vi "SimpleLiveAppBufferIndexScrollBar.vi"() -> ()   [LabVIEW 2018]
uses:
  D:/SVN/PM/sdk/AppSamples/LabVIEWSamples/trunk/Release/2018/Dependencies/PVCamNET.dll
  Dependencies/PVCamNET.dll
panel:
  out "Buffer Index":dbl
  in  "Scroll bar":i32(c297)
  out "Capturing":bool
  in  "Exposure Time":dbl
  out "Live":bool
  out "Camera Status":bool
  in  "Uninit":bool
  in  "Live stop":bool
  in  "Live start":bool
  in  "Init":bool
  # "SimpleLiveAppBufferIndexScrollBar.vi\n\nDescription:\nThis sample code lets the user use live mode in an event driven structure.\nWhen live mode is paused the user is able to scroll the bar to view images.\n\nSteps to run:\n1. Click \"Run\"\n2. Click \"Open\"\n3. Enter Exposure Time\n4. Click \"Live start\"\n5. Click \"Live stop\"\n6.  Scroll the scroll bar\n7. Click \"Close\""
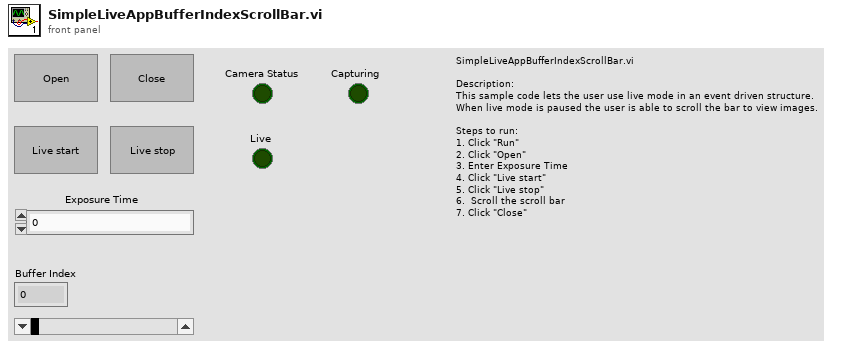
[diagram p1: front panel]
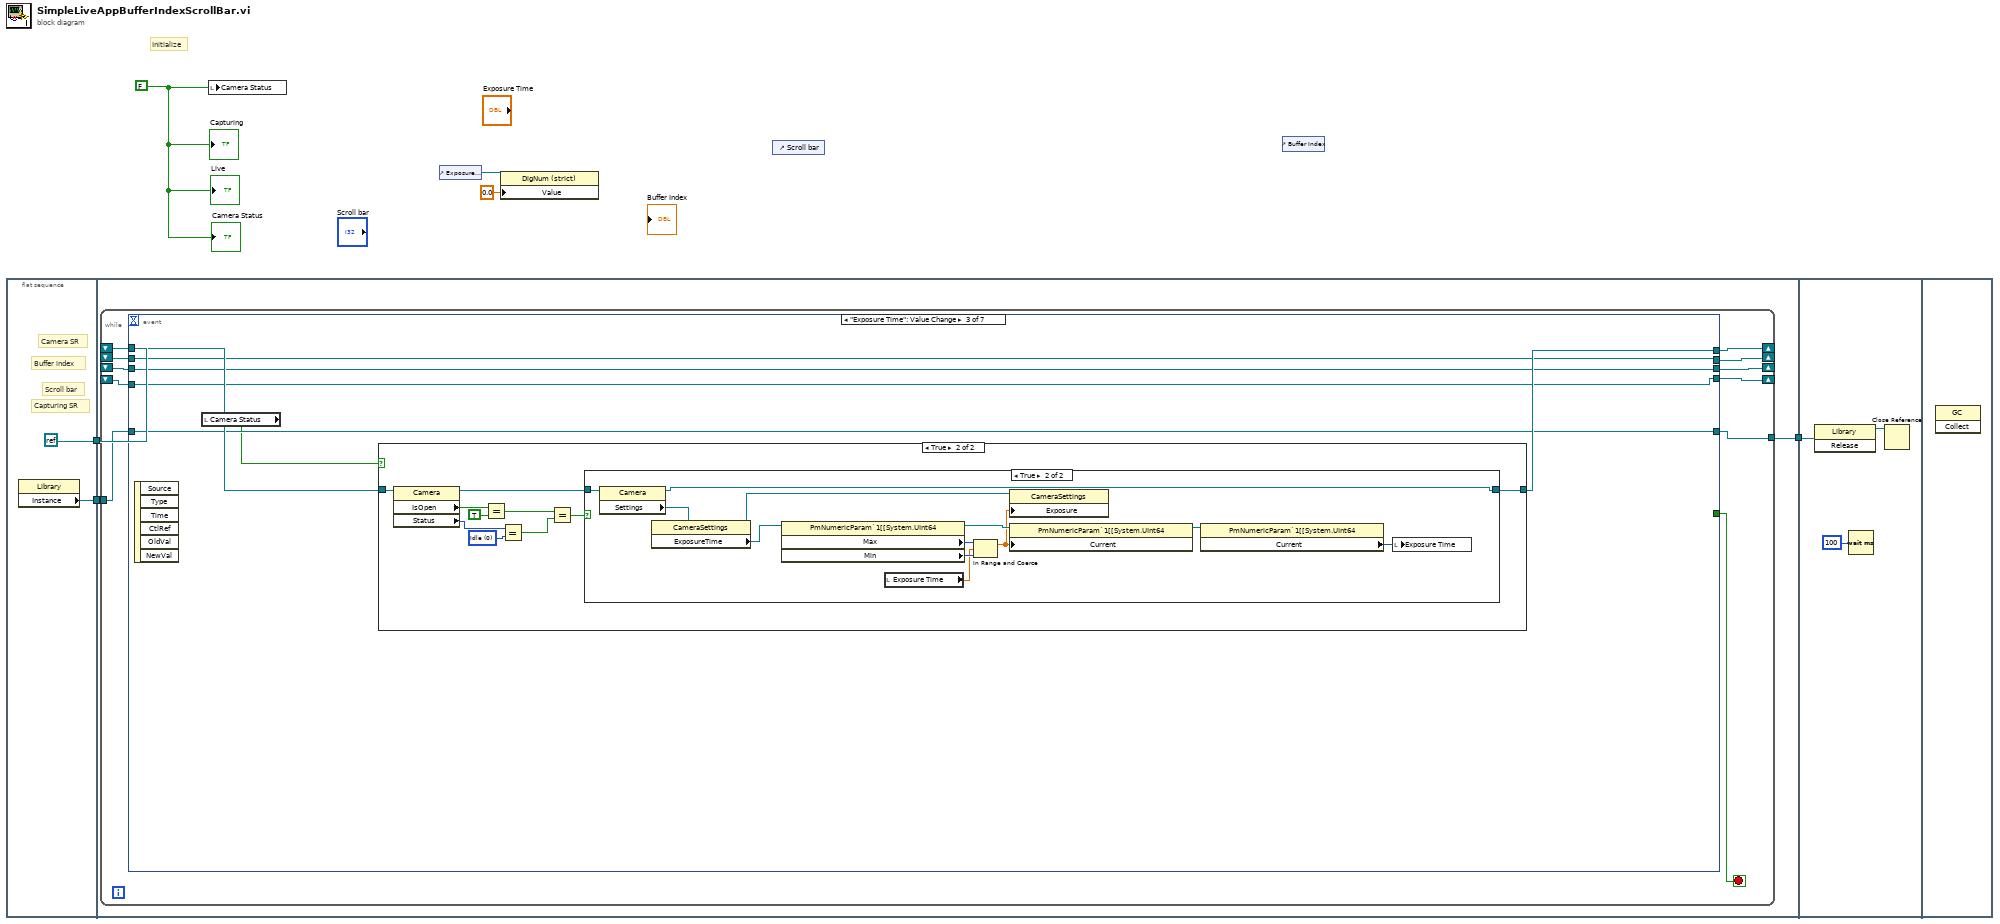
[diagram p0: block diagram]
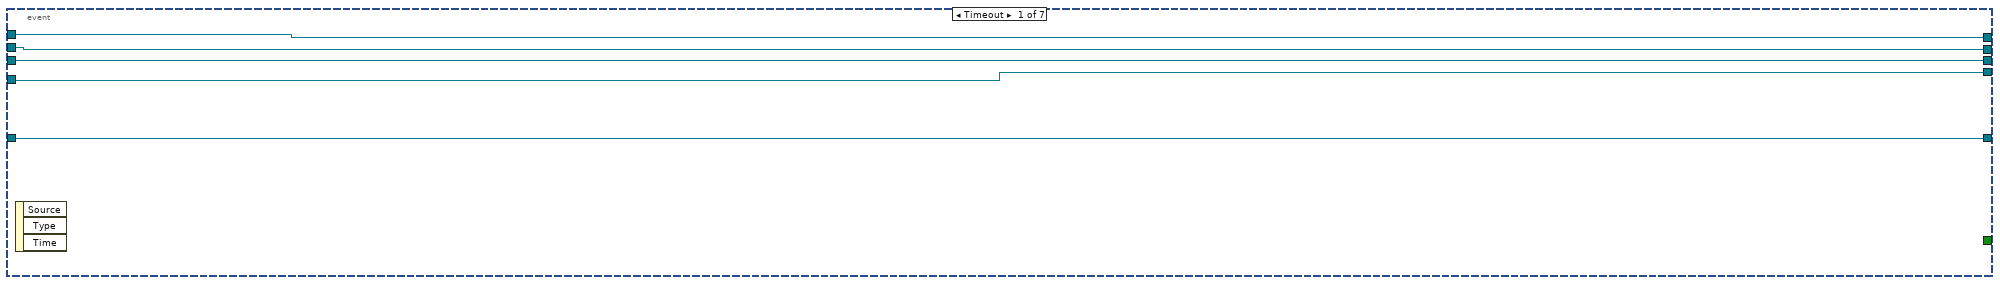
[diagram p2: hidden frame]
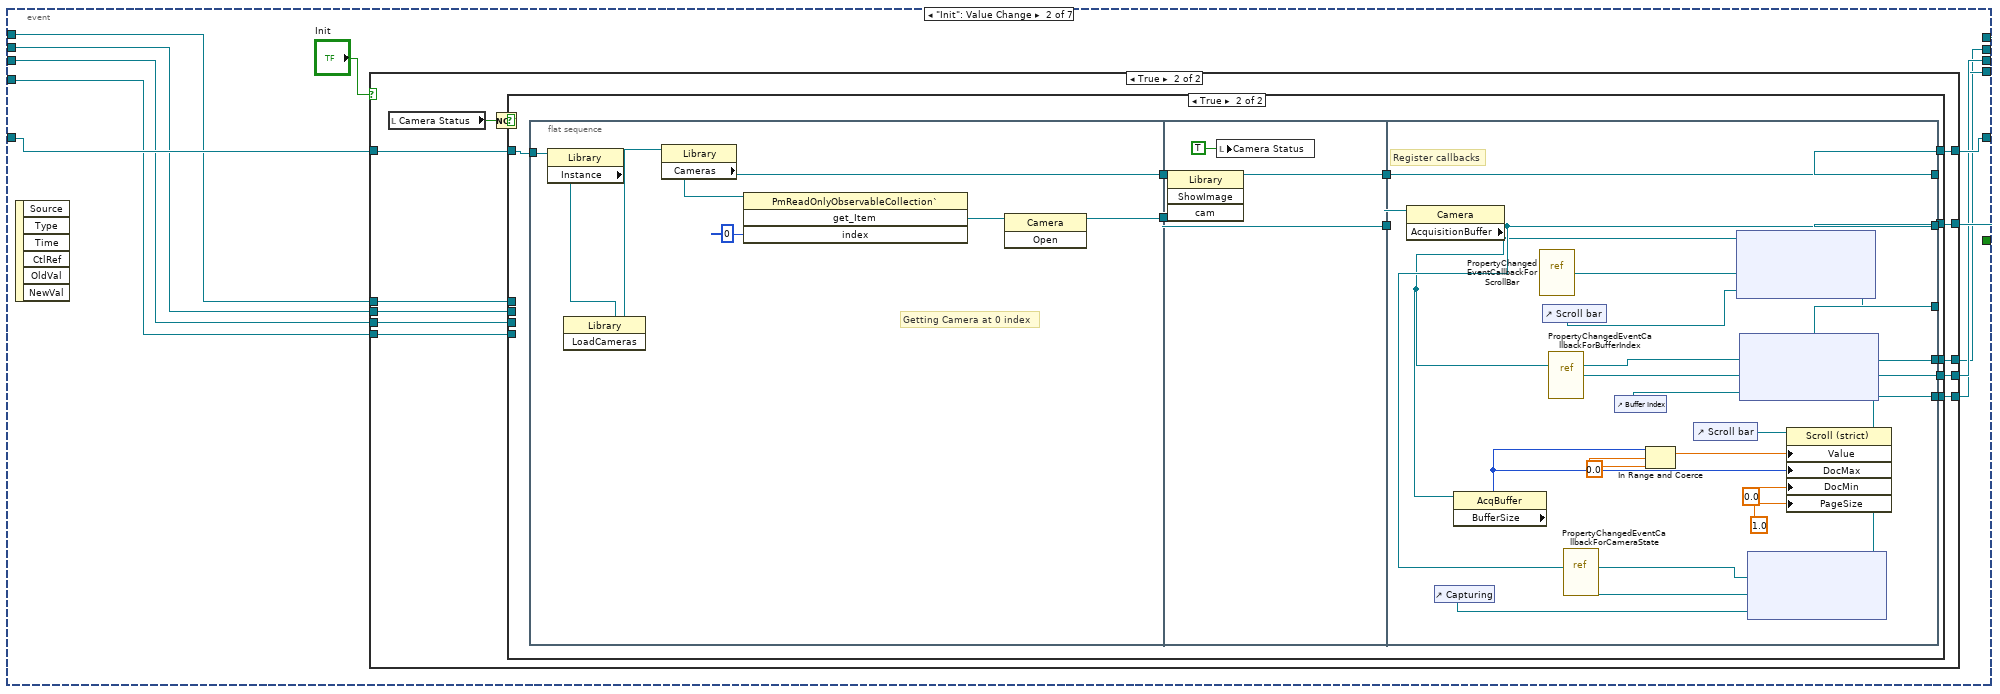
[diagram p3: hidden frame]
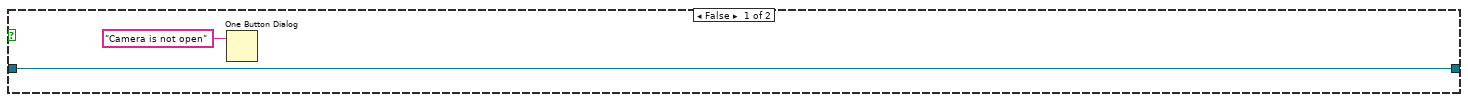
[diagram p6: hidden frame]
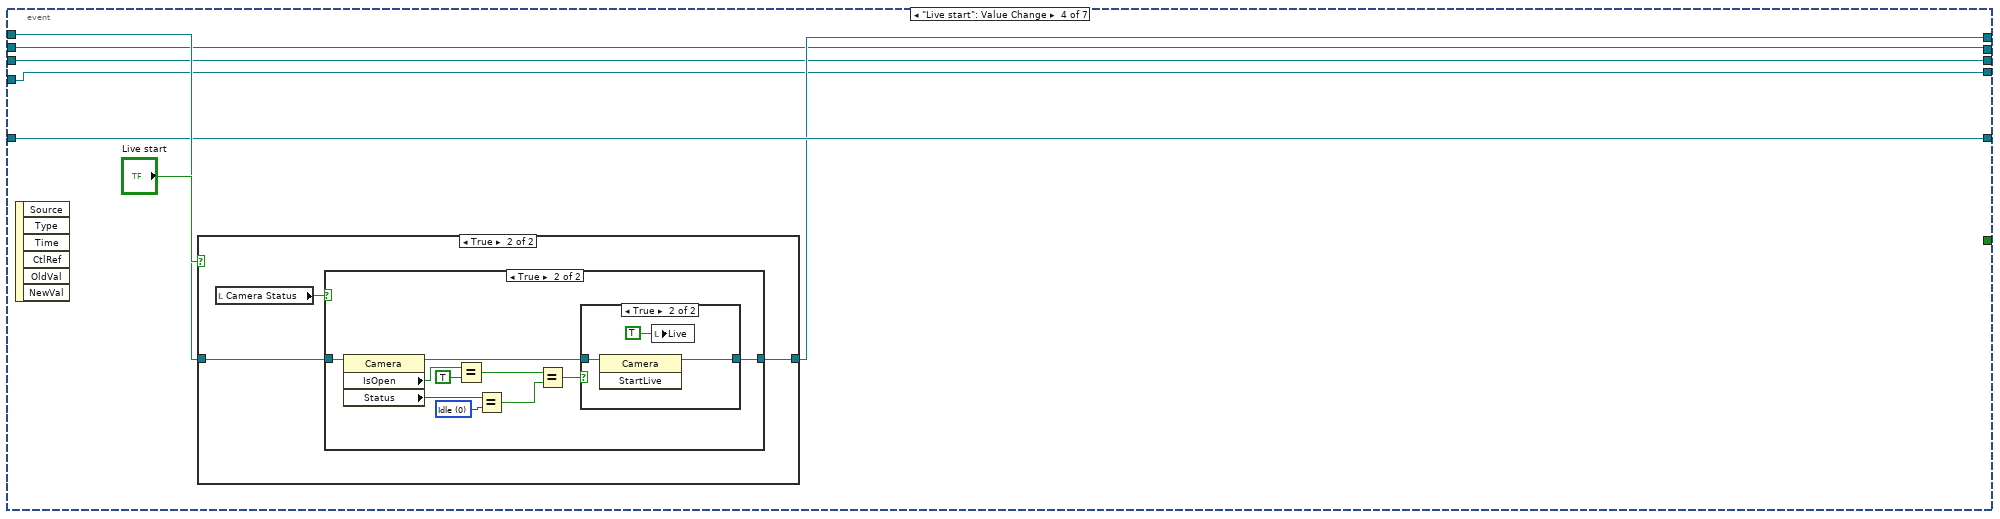
[diagram p8: hidden frame]
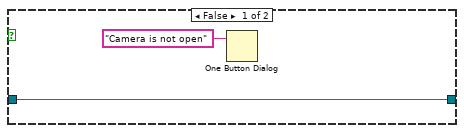
[diagram p10: hidden frame]
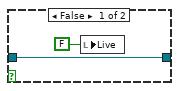
[diagram p11: hidden frame]
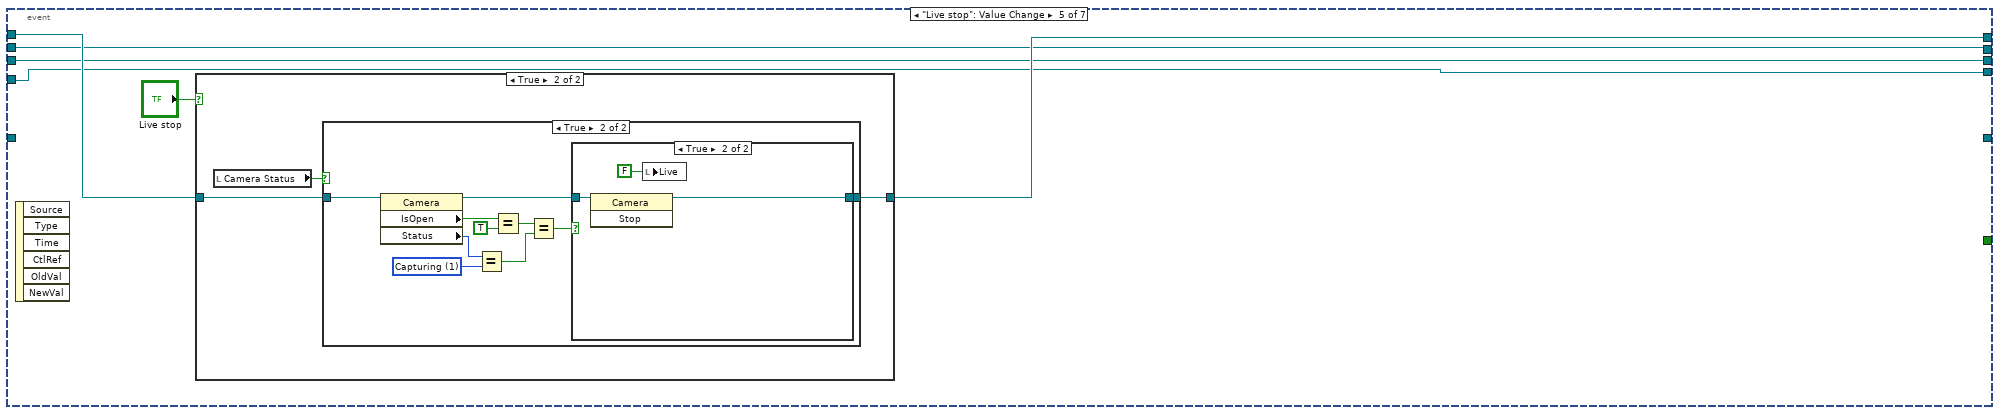
[diagram p12: hidden frame]
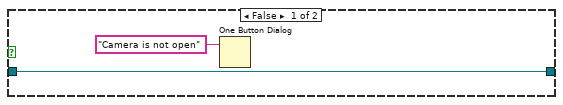
[diagram p14: hidden frame]
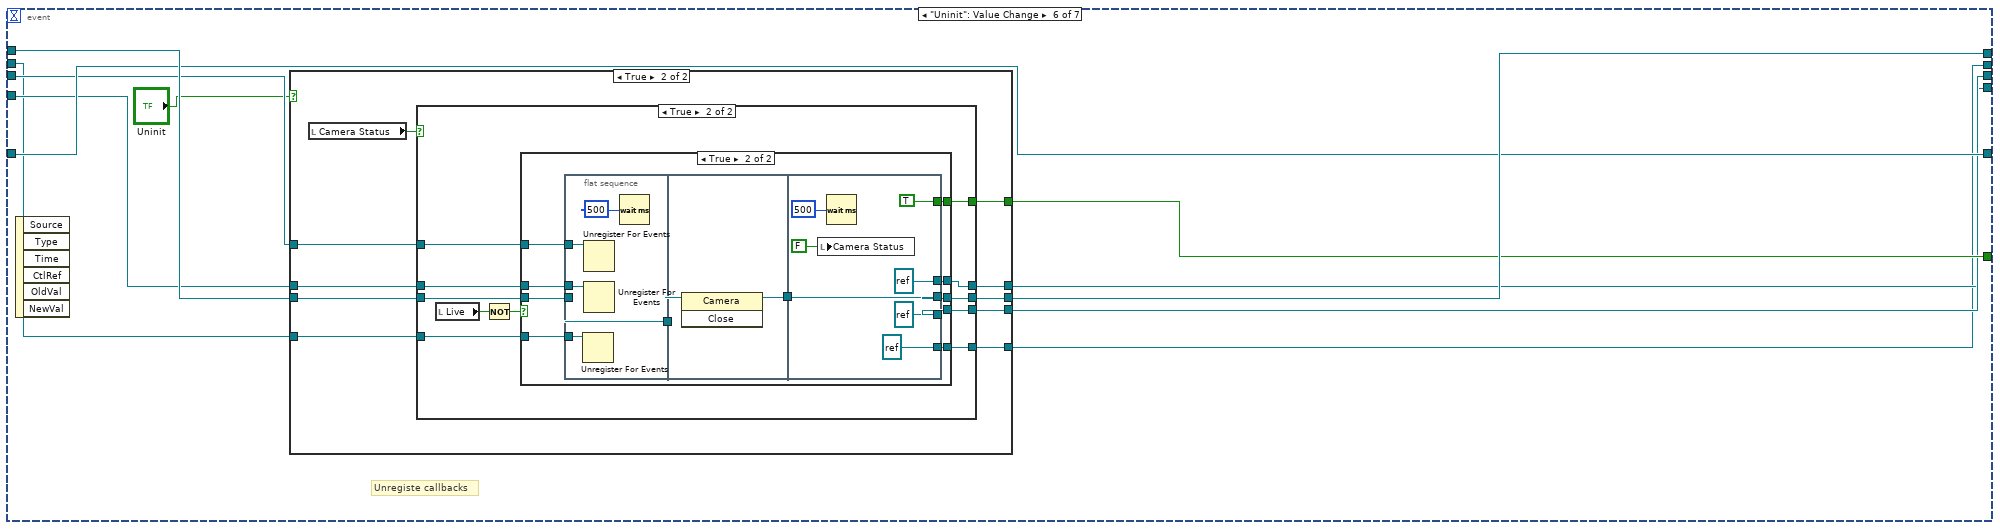
[diagram p16: hidden frame]
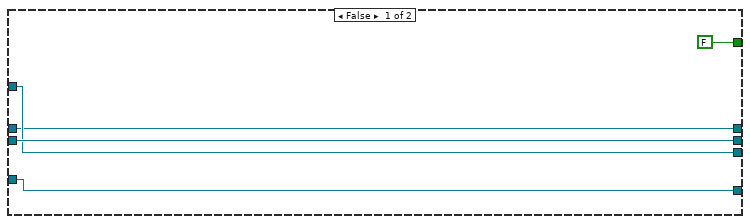
[diagram p17: hidden frame]
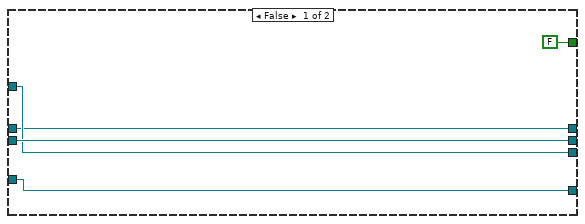
[diagram p18: hidden frame]
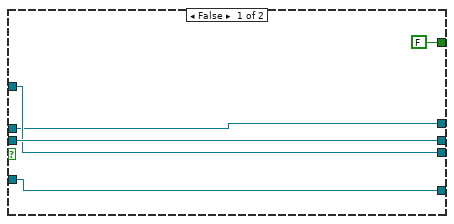
[diagram p19: hidden frame]
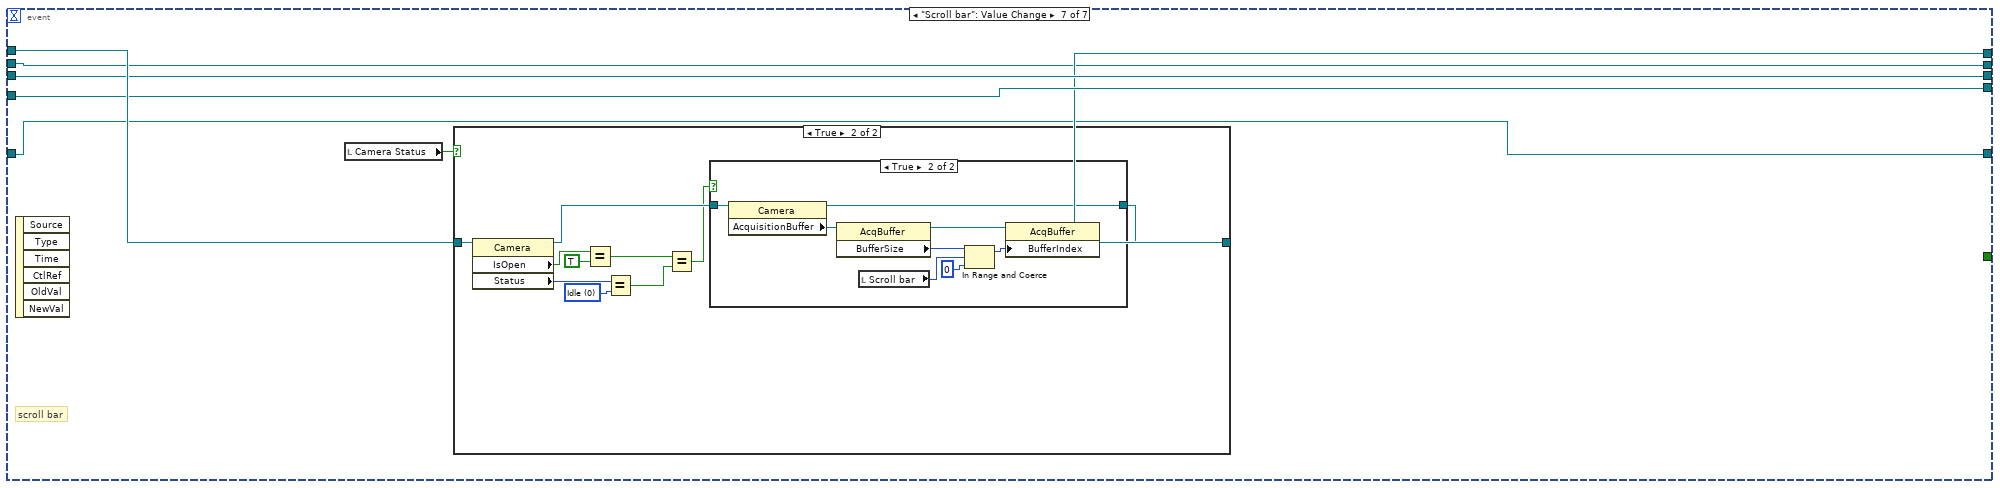
[diagram p20: hidden frame]
diagram:
  w3 = FALSE ("Histogram On/Off")
  # "Initialize"
  n1 = flat-sequence {
    tunnel: [w8] -> w6
    tunnel: [refnum<k0> refnum] -> w4
    tunnel: w6 -> [w11]
    tunnel: [w10] -> w5
    tunnel: w4 -> [w9]
    tunnel: w5 -> [w289]
    frame #0 {
      # "Buffer index"
      # "Capturing SR"
      # "Camera SR"
      # "Scroll bar"
      n2 = property class="Library"() -> ("Instance"=w8:refnum<k24>)  [unwired: 2 in, 2 out]
    }
    frame #1 {
      n3 = while {
        tunnel: w11 -> [w22]
        shift-right: [w21] -> _
        shift-left: w9 -> [w12]
        tunnel: [w20] -> w10
        shift-right: [w18] -> _
        shift-left: _ -> [w17]
        shift-right: [w16] -> _
        shift-left: _ -> [w15]
        shift-right: [w14] -> _
        shift-left: _ -> [w13]
        stop <- w19 stop-if-true
        n4 = event shown="[2] \"Exposure Time\": Value Change" {
          selector: _ -> [_ _ _ _ _ _ _]
          dyn-events: _ -> [_ _ _ _ _ _ _]
          timeout: _ -> [_ _ _ _ _ _ _]
          tunnel: w22 -> [w26 w38 w106 w138 _ w196 w262]
          tunnel: [w27 w37 w107 w137 w165 w197 w263] -> w21
          tunnel: [w26 w36 w106 w138 _ w196 w262] -> w20
          tunnel: w12 -> [w27 w35 w108 w139 w166 w198 w266]
          tunnel: [_ _ _ _ _ w195 _] -> w19
          tunnel: [w25 w33 w104 w136 w164 w193 w265] -> w18
          tunnel: w17 -> [w25 w29 w104 w136 w164 w194 w265]
          tunnel: [w24 w32 w103 w135 w163 w190 w264] -> w16
          tunnel: w15 -> [w24 w31 w103 w135 w163 w191 w264]
          tunnel: [w23 w30 w102 w134 w162 w189 w260] -> w14
          tunnel: w13 -> [w23 w28 w102 w134 w162 w188 w260]
          event Timeout {
            n5 = event-data() -> ()  [unwired: 1 in, 3 out]
          }
          event "Init": Value Change {
            n6 = event-data() -> ()  [unwired: 1 in, 6 out]
            n7 = case shown="True" "Init" {
              tunnel: w38 -> [w43 w55]
              tunnel: [w42 w54] -> w37
              tunnel: [w43 w53] -> w36
              tunnel: w35 -> [w42 w50]
              tunnel: [w41 w49] -> w33
              tunnel: w29 -> [w41 w48]
              tunnel: [w40 w47] -> w32
              tunnel: w31 -> [w40 w46]
              tunnel: [w39 w45] -> w30
              tunnel: w28 -> [w39 w44]
              frame False {
              }
              frame True {
                n8 = local read "Camera Status"() -> (w52:bool)
                n9 = Not(x=w52) -> (.not. x?=w51:bool)
                n10 = case shown="True" w51 {
                  tunnel: w55 -> [w59 w68]
                  tunnel: [w60 w67] -> w54
                  tunnel: [w59 w66] -> w53
                  tunnel: w50 -> [w60 _]
                  tunnel: [w58 w63] -> w49
                  tunnel: w48 -> [w58 _]
                  tunnel: [w57 w62] -> w47
                  tunnel: w46 -> [w57 _]
                  tunnel: [w56 w61] -> w45
                  tunnel: w44 -> [w56 _]
                  frame False {
                  }
                  frame True {
                    n11 = flat-sequence {
                      tunnel: w68 -> [w73]
                      tunnel: [w75] -> w70
                      tunnel: [w74] -> w69
                      tunnel: w70 -> [w81]
                      tunnel: w69 -> [w82]
                      tunnel: [w82] -> w65
                      tunnel: [w80] -> w64
                      tunnel: [w101] -> w66
                      tunnel: [w98] -> w67
                      tunnel: w65 -> [w100]
                      tunnel: w64 -> [w101]
                      tunnel: [w94] -> w63
                      tunnel: [w97] -> w62
                      tunnel: [w93] -> w61
                      frame #0 {
                        # "Getting Camera at 0 index"
                        n12 = property class="Library"(reference=w73) -> ("Instance"=w72:refnum<k24>)  [unwired: 1 in, 2 out]
                        n13 = invoke class="Library" method="LoadCameras"(reference=w72) -> (reference out=w71:refnum<k24>)  [unwired: 2 in, 2 out]
                        n14 = property class="Library"(reference=w71) -> (reference out=w75:refnum<k24>, "Cameras"=w78:refnum<k24>)  [unwired: 1 in, 1 out]
                        n15 = invoke class="PmReadOnlyObservableCollection`" method="get_Item"(reference=w78, "index"=0) -> ("get_Item"=w76:refnum<k24>)  [unwired: 2 in, 3 out]
                        n16 = invoke class="Camera" method="Open"(reference=w76) -> (reference out=w74:refnum<k24>)  [unwired: 2 in, 2 out]
                      }
                      frame #1 {
                        n17 = invoke class="Library" method="ShowImage"(reference=w81, "cam"=w82) -> (reference out=w80:refnum<k24>)  [unwired: 2 in, 3 out]
                        n18 = local write "Camera Status"(TRUE ("Camera Status")) -> ()
                      }
                      frame #2 {
                        w85 = 0.0 ("upper limit")
                        # "Register callbacks"
                        n19 = property class="Camera"(reference=w100) -> (reference out=w98:refnum<k24>, "AcquisitionBuffer"=w90:refnum<k24>)  [unwired: 1 in, 1 out]
                        n20 = control-ref of="Capturing"() -> (w99:refnum<vi>)
                        n21 = property class="AcqBuffer"(reference=w90) -> ("BufferSize"=w86:u32)  [unwired: 1 in, 2 out]
                        n22 = vi-ref "PropertyChangedEventCallbackForScrollBar.vi"() -> ("vi reference"=w87:refnum<vi>)
                        n23 = control-ref of="Scroll bar"() -> (w88:refnum<vi>)
                        n24 = vi-ref "PropertyChangedEventCallbackForBufferIndex.vi"() -> ("vi reference"=w91:refnum<vi>)
                        n25 = vi-ref "PropertyChangedEventCallbackForCameraState.vi"() -> ("vi reference"=w96:refnum<vi>)
                        n26 = control-ref of="Buffer Index"() -> (w92:refnum<vi>)
                        n27 = In Range and Coerce(upper limit=w86, x=w85, lower limit=w85) -> (coerced(x)=w89:dbl)  [unwired: 1 out]
                        n28 = control-ref of="Scroll bar"() -> (w95:refnum<vi>)
                        n29 = node(w90, w87, w88) -> (w94:refnum<k27>)  [unwired: 2 in, 1 out]
                        n30 = node(w90, w91, w92) -> (w93:refnum<k27>)  [unwired: 2 in, 1 out]
                        n31 = node(w98, w96, w99) -> (w97:refnum<k27>)  [unwired: 2 in, 1 out]
                        n32 = property class="Scroll (strict)"(reference=w95, "Value"=w89, "DocMax"=w86, "DocMin"=0.0 ("upper limit"), "PageSize"=1.0 ("Page Size")) -> ()  [unwired: 1 in, 2 out]
                      }
                    }
                  }
                }
              }
            }
          }
          event "Exposure Time": Value Change {
            n33 = event-data() -> ()  [unwired: 1 in, 6 out]
            n34 = local read "Camera Status"() -> (w105:bool)
            n35 = case shown="True" w105 {
              tunnel: w108 -> [w110 w114]
              tunnel: [w110 w111] -> w107
              frame False {
                n36 = One Button Dialog(message="Camera is not open") -> ()  [unwired: 1 in, 1 out]
              }
              frame True {
                w119 = 0 items=["Idle", "Capturing"] ("Status")
                n37 = property class="Camera"(reference=w114) -> (reference out=w112:refnum<k24>, "IsOpen"=w118:bool, "Status"=w120:i32)  [unwired: 1 in, 1 out]
                n38 = Equal?(x=w118, y=TRUE) -> (x = y?=w116:bool)
                n39 = Equal?(x=w120, y=w119) -> (x = y?=w115:bool)
                n40 = Equal?(x=w116, y=w115) -> (x = y?=w113:bool)
                n41 = case shown="True" w113 {
                  tunnel: w112 -> [w121 w133]
                  tunnel: [w121 w125] -> w111
                  frame False {
                  }
                  frame True {
                    n42 = property class="Camera"(reference=w133) -> (reference out=w125:refnum<k24>, "Settings"=w124:refnum<k24>)  [unwired: 1 in, 1 out]
                    n43 = property class="CameraSettings"(reference=w124) -> (reference out=w122:refnum<k24>, "ExposureTime"=w123:refnum<k24>)  [unwired: 1 in, 1 out]
                    n44 = property class="PmNumericParam`1[[System.UInt64"(reference=w123) -> (reference out=w130:refnum<k24>, "Max"=w132:u64, "Min"=w131:u64)  [unwired: 1 in, 1 out]
                    n45 = local read "Exposure Time"() -> (w127:dbl)
                    n46 = In Range and Coerce(upper limit=w132, x=w127, lower limit=w131) -> (coerced(x)=w128:dbl)  [unwired: 1 out]
                    n47 = property class="CameraSettings"(reference=w122, "Exposure"=w128) -> ()  [unwired: 1 in, 2 out]
                    n48 = property class="PmNumericParam`1[[System.UInt64"(reference=w130, "Current"=w128) -> (reference out=w129:refnum<k24>)  [unwired: 1 in, 1 out]
                    n49 = property class="PmNumericParam`1[[System.UInt64"(reference=w129) -> ("Current"=w126:u64)  [unwired: 1 in, 2 out]
                    n50 = local write "Exposure Time"(w126) -> ()
                  }
                }
              }
            }
          }
          event "Live start": Value Change {
            n51 = event-data() -> ()  [unwired: 1 in, 6 out]
            n52 = case shown="True" "Live start" {
              tunnel: w139 -> [w141 w144]
              tunnel: [w141 w143] -> w137
              frame False {
              }
              frame True {
                n53 = local read "Camera Status"() -> (w142:bool)
                n54 = case shown="True" w142 {
                  tunnel: w144 -> [w145 w150]
                  tunnel: [w145 w148] -> w143
                  frame False {
                    n55 = One Button Dialog(message="Camera is not open") -> ()  [unwired: 1 in, 1 out]
                  }
                  frame True {
                    w155 = 0 items=["Idle", "Capturing"] ("Status")
                    n56 = property class="Camera"(reference=w150) -> (reference out=w149:refnum<k24>, "IsOpen"=w154:bool, "Status"=w156:i32)  [unwired: 1 in, 1 out]
                    n57 = Equal?(x=w154, y=TRUE) -> (x = y?=w152:bool)
                    n58 = Equal?(x=w156, y=w155) -> (x = y?=w151:bool)
                    n59 = Equal?(x=w152, y=w151) -> (x = y?=w147:bool)
                    n60 = case shown="True" w147 {
                      tunnel: w149 -> [w158 w159]
                      tunnel: [w158 w160] -> w148
                      frame False {
                        n61 = local write "Live"(FALSE ("Live 2")) -> ()
                      }
                      frame True {
                        n62 = invoke class="Camera" method="StartLive"(reference=w159) -> (reference out=w160:refnum<k24>)  [unwired: 2 in, 2 out]
                        n63 = local write "Live"(TRUE ("Live")) -> ()
                      }
                    }
                  }
                }
              }
            }
          }
          event "Live stop": Value Change {
            n64 = event-data() -> ()  [unwired: 1 in, 6 out]
            n65 = case shown="True" "Live stop" {
              tunnel: w166 -> [w168 w171]
              tunnel: [w168 w170] -> w165
              frame False {
              }
              frame True {
                n66 = local read "Camera Status"() -> (w169:bool)
                n67 = case shown="True" w169 {
                  tunnel: w171 -> [w173 w183]
                  tunnel: [w173 w180] -> w170
                  frame False {
                    n68 = One Button Dialog(message="Camera is not open") -> ()  [unwired: 1 in, 1 out]
                  }
                  frame True {
                    w178 = 1 items=["Idle", "Capturing"] ("Status")
                    n69 = property class="Camera"(reference=w183) -> (reference out=w181:refnum<k24>, "IsOpen"=w177:bool, "Status"=w179:i32)  [unwired: 1 in, 1 out]
                    n70 = Equal?(x=w179, y=w178) -> (x = y?=w174:bool)
                    n71 = Equal?(x=w177, y=TRUE) -> (x = y?=w175:bool)
                    n72 = Equal?(x=w175, y=w174) -> (x = y?=w182:bool)
                    n73 = case shown="True" w182 {
                      tunnel: w181 -> [w184 w187]
                      tunnel: [w184 w186] -> w180
                      frame False {
                      }
                      frame True {
                        n74 = invoke class="Camera" method="Stop"(reference=w187) -> (reference out=w186:refnum<k24>)  [unwired: 2 in, 2 out]
                        n75 = local write "Live"(FALSE ("Live 2")) -> ()
                      }
                    }
                  }
                }
              }
            }
          }
          event "Uninit": Value Change {
            # "Unregiste callbacks"
            n76 = event-data() -> ()  [unwired: 1 in, 6 out]
            n77 = case shown="True" "Uninit" {
              tunnel: w198 -> [w203 w213]
              tunnel: [w203 w212] -> w197
              tunnel: [FALSE ("Camera Status") w210] -> w195
              tunnel: w194 -> [w201 w209]
              tunnel: [w201 w208] -> w193
              tunnel: w191 -> [w200 w207]
              tunnel: [w200 w206] -> w190
              tunnel: [w199 w205] -> w189
              tunnel: w188 -> [w199 w204]
              frame False {
              }
              frame True {
                n78 = local read "Camera Status"() -> (w211:bool)
                n79 = case shown="True" w211 {
                  tunnel: w213 -> [w218 w229]
                  tunnel: [w218 w228] -> w212
                  tunnel: [FALSE ("Camera Status") w227] -> w210
                  tunnel: w209 -> [w216 w224]
                  tunnel: [w216 w223] -> w208
                  tunnel: w207 -> [w215 w222]
                  tunnel: [w215 w221] -> w206
                  tunnel: [w214 w220] -> w205
                  tunnel: w204 -> [w214 w219]
                  frame False {
                  }
                  frame True {
                    n80 = local read "Live"() -> (w225:bool)
                    n81 = Not(x=w225) -> (.not. x?=w226:bool)
                    n82 = case shown="True" w226 {
                      tunnel: w229 -> [w234 w244]
                      tunnel: [w234 w243] -> w228
                      tunnel: [FALSE ("Camera Status") w242] -> w227
                      tunnel: w224 -> [w232 w240]
                      tunnel: [w232 w239] -> w223
                      tunnel: w222 -> [w231 w238]
                      tunnel: [w231 w237] -> w221
                      tunnel: [w230 w236] -> w220
                      tunnel: w219 -> [w230 w235]
                      frame False {
                      }
                      frame True {
                        n83 = flat-sequence {
                          tunnel: w244 -> [w250]
                          tunnel: [w250] -> w241
                          tunnel: w240 -> [w249]
                          tunnel: w238 -> [w247]
                          tunnel: w235 -> [w246]
                          tunnel: [w251] -> w245
                          tunnel: w241 -> [w252]
                          tunnel: [w259] -> w243
                          tunnel: w245 -> [w259]
                          tunnel: [TRUE ("Camera Status")] -> w242
                          tunnel: [refnum<k27> refnum ("Event Callback")] -> w239
                          tunnel: [refnum<k27> refnum ("Event Callback")] -> w237
                          tunnel: [refnum<k27> refnum ("Event Callback")] -> w236
                          frame #0 {
                            n84 = Unregister For Events(event registration refnum=w246) -> ()  [unwired: 1 in, 1 out]
                            n85 = Unregister For Events(event registration refnum=w249) -> ()  [unwired: 1 in, 1 out]
                            n86 = Unregister For Events(event registration refnum=w247) -> ()  [unwired: 1 in, 1 out]
                            n87 = Wait (ms)(milliseconds to wait=u32 500) -> ()  [unwired: 1 out]
                          }
                          frame #1 {
                            n88 = invoke class="Camera" method="Close"(reference=w252) -> (reference out=w251:refnum<k24>)  [unwired: 2 in, 2 out]
                          }
                          frame #2 {
                            n89 = local write "Camera Status"(FALSE ("Camera Status")) -> ()
                            n90 = Wait (ms)(milliseconds to wait=u32 500) -> ()  [unwired: 1 out]
                          }
                        }
                      }
                    }
                  }
                }
              }
            }
          }
          event "Scroll bar": Value Change {
            # "scroll bar"
            n91 = event-data() -> ()  [unwired: 1 in, 6 out]
            n92 = local read "Camera Status"() -> (w261:bool)
            n93 = case shown="True" w261 {
              tunnel: w266 -> [w267 w272]
              tunnel: [w267 w270] -> w263
              frame False {
                n94 = One Button Dialog(message="Camera is not open") -> ()  [unwired: 1 in, 1 out]
              }
              frame True {
                w277 = 0 items=["Idle", "Capturing"] ("Status")
                n95 = property class="Camera"(reference=w272) -> (reference out=w271:refnum<k24>, "IsOpen"=w276:bool, "Status"=w278:i32)  [unwired: 1 in, 1 out]
                n96 = Equal?(x=w276, y=TRUE) -> (x = y?=w274:bool)
                n97 = Equal?(x=w278, y=w277) -> (x = y?=w273:bool)
                n98 = Equal?(x=w274, y=w273) -> (x = y?=w269:bool)
                n99 = case shown="True" w269 {
                  tunnel: w271 -> [w279 w287]
                  tunnel: [w279 w286] -> w270
                  frame False {
                  }
                  frame True {
                    n100 = property class="Camera"(reference=w287) -> (reference out=w286:refnum<k24>, "AcquisitionBuffer"=w284:refnum<k24>)  [unwired: 1 in, 1 out]
                    n101 = property class="AcqBuffer"(reference=w284) -> (reference out=w280:refnum<k24>, "BufferSize"=w283:u32)  [unwired: 1 in, 1 out]
                    n102 = local read "Scroll bar"() -> (w285:i32)
                    n103 = In Range and Coerce(upper limit=w283, x=w285, lower limit=0) -> (coerced(x)=w281:u32)  [unwired: 1 out]
                    n104 = property class="AcqBuffer"(reference=w280, "BufferIndex"=w281) -> ()  [unwired: 1 in, 2 out]
                  }
                }
              }
            }
          }
        }
      }
    }
    frame #2 {
      n105 = invoke class="Library" method="Release"(reference=w289) -> (reference out=w290:refnum<k24>)  [unwired: 2 in, 2 out]
      n106 = Wait (ms)(milliseconds to wait=u32 100) -> ()  [unwired: 1 out]
      n107 = Close Reference(reference=w290) -> ()  [unwired: 1 in, 1 out]
    }
    frame #3 {
      n108 = invoke class="GC" method="Collect"() -> ()  [unwired: 3 in, 3 out]
    }
  }
  n109 = local write "Camera Status"(w3) -> ()
  n110 = control-ref of="Exposure Time"() -> (w2:refnum<vi>)
  n111 = property class="DigNum (strict)"(reference=w2, "Value"=0.0) -> ()  [unwired: 1 in, 2 out]
  n112 = control-ref of="Scroll bar"() -> ()  [unwired: 1 out]
  n113 = control-ref of="Buffer Index"() -> ()  [unwired: 1 out]
  "Camera Status" <- w3
  "Live" <- w3
  "Capturing" <- w3
